vi "ep_THDS THDG.vi"(11 "Array":dbl[](array[numeric])) -> (3 "Numeric":dbl)   [LabVIEW 2011, in "NI_EP_Power Quality.lvlib"]
uses:
  <vilib>/addons/Electrical Power/PQ/NI_EP_Power Quality.lvlib
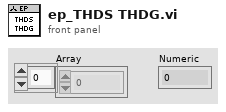
[diagram p1: front panel]
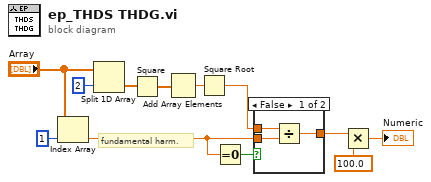
[diagram p0: block diagram]
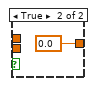
[diagram p2: hidden frame]
diagram:
  # "fundamental harm."
  n1 = Index Array(array="Array", index=1) -> (element=w1:dbl)
  n2 = Split 1D Array(array="Array", index=2) -> (second subarray=w10:dbl[])  [unwired: 1 out]
  n3 = Square(x=w10) -> (x^2=w11:dbl[])
  n4 = Add Array Elements(numeric array=w11) -> (sum=w12:dbl)
  n5 = Square Root(x=w12) -> (sqrt(x)=w3:dbl)
  n6 = Equal To 0?(x=w1) -> (x = 0?=w5:bool)
  n7 = case shown="False" w5 {
    tunnel: w1 -> [w14 _]
    tunnel: [w13 0.0 ("t")] -> w2
    tunnel: w3 -> [w15 _]
    frame False {
      n8 = Divide(x=w15, y=w14) -> (x/y=w13:dbl)
    }
    frame True {
    }
  }
  n9 = Multiply(x=w2, y=100.0) -> (x*y=→"Numeric":dbl)
